vi "rad2deg (SubVI).vi"(1 "Angle (rad)":dbl) -> (0 "Angle(deg)":dbl)   [LabVIEW 2010]
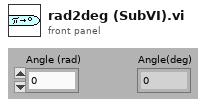
[diagram p1: front panel]
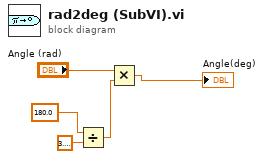
[diagram p0: block diagram]
diagram:
  n1 = Divide(x=180.0 ("y"), y=3.141592653589793) -> (x/y=w2:dbl)
  n2 = Multiply(x="Angle (rad)", y=w2) -> (x*y=→"Angle(deg)":dbl)
